vi "Global_Next_Scan_Position.vi"() -> ()   [LabVIEW 2018]
panel:
  in  "XAS(f) / XPS(t)":bool
  in  "verfluchter Kackdreck":bool
  in  "MM Scan":u16
  in  "Next Scan Pos":i32[](array[numeric])
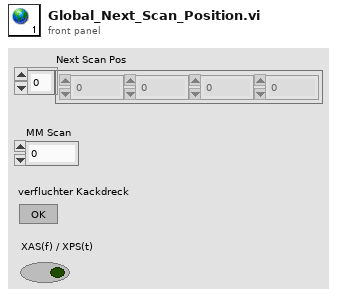
[diagram p1: front panel]
diagram:
